vi "Get Actual Monitor #.vi"(6 "Monitor Order Override (3,2,1,4)":i8[](array[numeric])=[3, 2, 1, 4], 11 "Requested Monitor (1,2,3,4...)":i8) -> (2 "Enough Monitors?":bool, 3 "Actual Monitor Index out":i8)   [LabVIEW 2018]
doc: "Uses the monitor bounds to get the actual monitor number (index) starting at index 1.\n\nIt sorts first from left to right.\nIf any monitors are directly on top of each other, it sorts those monitors from top to bottom."
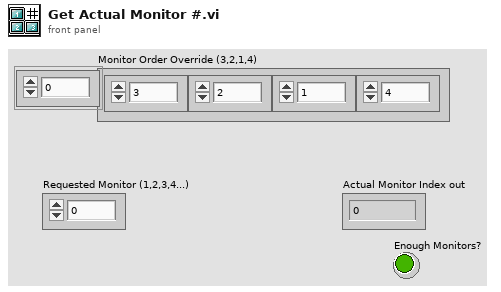
[diagram p1: front panel]
types:
  T1 = typedef "LVAllMonitorsDisplayTypeDef.ctl" = cluster{"Bounds":cluster{"Left":i16, "Top":i16, "Right":i16, "Bottom":i16}, "Depth":i16}[]
  T2 = cluster{"Left":i16, "Monitor Info":cluster{"Bounds":cluster{"Left":i16, "Top":i16, "Right":i16, "Bottom":i16}, "Depth":i16}, "Original Index":i32}
  T3 = cluster{"Left":i16, "Monitor Info":cluster{"Bounds":cluster{"Left":i16, "Top":i16, "Right":i16, "Bottom":i16}, "Depth":i16}, "Original Index":i32}[]
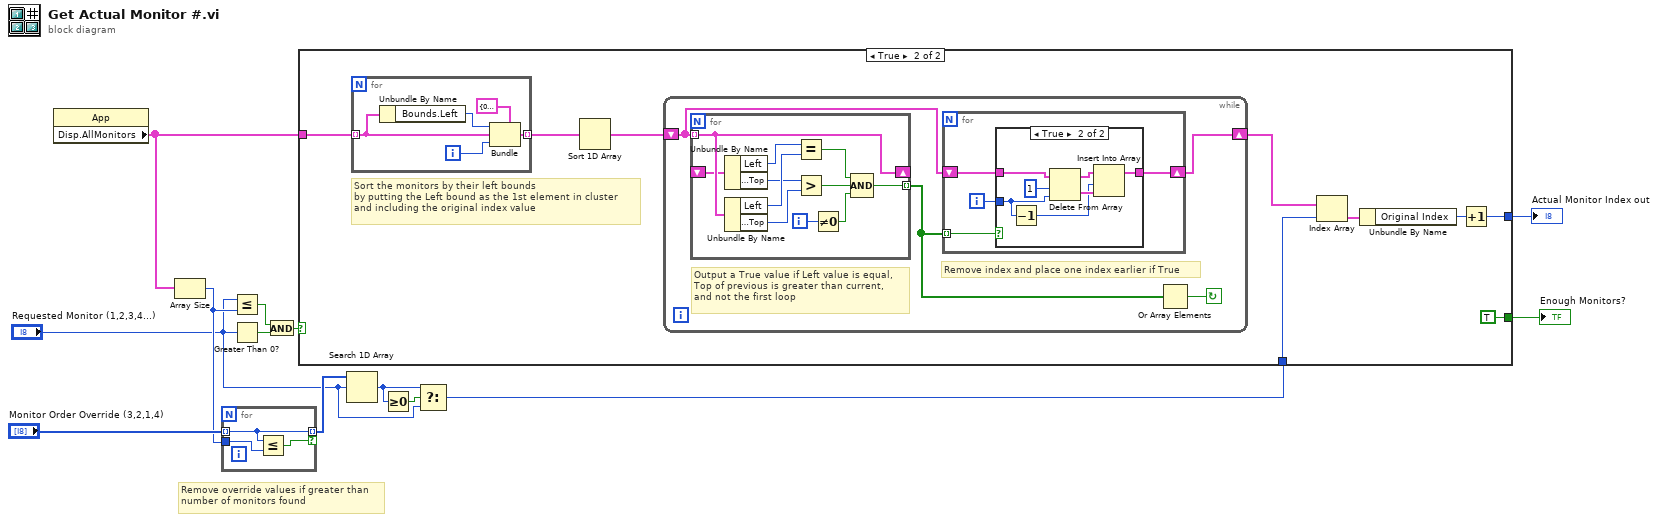
[diagram p0: block diagram]
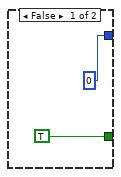
[diagram p2: hidden frame]
diagram:
  # "Remove override values if greater than\nnumber of monitors found"
  n1 = property class="App"() -> ("Disp.AllMonitors"=w1:T1)  [unwired: 2 in, 2 out]
  n2 = Array Size(array=w1) -> (size(s)=w5:i32)
  n3 = for {
    tunnel: "Monitor Order Override (3,2,1,4)" -> [w16] mode=indexing
    tunnel: [w16] -> w4 mode=indexing if=w14
    tunnel: w5 -> [w15]
    n4 = Less Or Equal?(x=w16, y=w15) -> (x <= y?=w14:bool)
  }
  n5 = Less Or Equal?(x="Requested Monitor (1,2,3,4...)", y=w5) -> (x <= y?=w11:bool)
  n6 = Greater Than 0?(x="Requested Monitor (1,2,3,4...)") -> (x > 0?=w9:bool)
  n7 = And(x=w11, y=w9) -> (x .and. y?=w10:bool)
  n8 = Search 1D Array(1D array=w4, element="Requested Monitor (1,2,3,4...)") -> (index of element=w8:i32)  [unwired: 1 in]
  n9 = Greater Or Equal To 0?(x=w8) -> (x >= 0?=w6:bool)
  n10 = Select(t=w8, s=w6, f="Requested Monitor (1,2,3,4...)") -> (s? t:f=w7:i32)
  n11 = case shown="True" w10 {
    tunnel: w1 -> [_ w25]
    tunnel: [0 w21] -> w12
    tunnel: w7 -> [_ w20]
    tunnel: [TRUE TRUE] -> w3
    frame False {
    }
    frame True {
      # "Sort the monitors by their left bounds\nby putting the Left bound as the 1st element in cluster\nand including the original index value"
      n12 = for {
        tunnel: w25 -> [w58] mode=indexing
        tunnel: [w57] -> w27 mode=indexing
        i -> [w56]
        n13 = Unbundle By Name(w58) -> ("Bounds.Left"=w59:i16)
        n14 = Bundle(cluster=T2 {"Left"=0, "Monitor Info"={"Bounds"={"Left"=0, "Top"=0, "Right"=0, "Bottom"=0}, "Depth"=0}, "Original Index"=0} ("output cluster"), "Left"=w59, "Monitor Info"=w58, "Original Index"=w56) -> (w57:T2)
      }
      n15 = Sort 1D Array(array=w27) -> (sorted array=w26:T3)
      n16 = while {
        shift-right: [w30] -> w24
        shift-left: w26 -> [w31]
        stop <- w28 continue-if-true
        # "Remove index and place one index earlier if True"
        # "Output a True value if Left value is equal,\nTop of previous is greater than current,\nand not the first loop"
        n17 = for {
          tunnel: w31 -> [w53] mode=indexing
          shift-right: [w53] -> _
          shift-left: _ -> [w52]
          tunnel: [w46] -> w29 mode=indexing
          i -> [w54]
          n18 = Unbundle By Name(w52) -> ("Left"=w50:i16, "Monitor Info.Bounds.Top"=w44:i16)
          n19 = Unbundle By Name(w53) -> ("Left"=w51:i16, "Monitor Info.Bounds.Top"=w45:i16)
          n20 = Equal?(x=w50, y=w51) -> (x = y?=w49:bool)
          n21 = Greater?(x=w44, y=w45) -> (0:w48:bool)
          n22 = Not Equal To 0?(x=w54) -> (x != 0?=w47:bool)
          n23 = Compound Arithmetic op=AND(w49, w48, w47) -> (w46:bool)
        }
        n24 = for {
          shift-right: [w33] -> w30
          shift-left: w31 -> [w35]
          tunnel: w29 -> [w34] mode=indexing
          i -> [w32]
          n25 = case shown="True" w34 {
            tunnel: w35 -> [w36 w43]
            tunnel: [w36 w40] -> w33
            tunnel: w32 -> [_ w38]
            frame False {
            }
            frame True {
              n26 = Decrement(x=w38) -> (x-1=w37:i32)
              n27 = Delete From Array(array=w43, length=1, index=w38) -> (deleted portion=w39:T3, array with subset deleted=w41:T3)
              n28 = Insert Into Array(array=w41, index=w37, new element=w39) -> (w40:T3)
            }
          }
        }
        n29 = Or Array Elements(Boolean array=w29) -> (logical OR=w28:bool)
      }
      n30 = Index Array(array=w24, index=w20) -> (element=w23:T2)
      n31 = Unbundle By Name(w23) -> ("Original Index"=w22:i32)
      n32 = Increment(x=w22) -> (x+1=w21:i32)
    }
  }
  "Enough Monitors?" <- w3
  "Actual Monitor Index out" <- w12
